vi "DiffIO PWM Disable.vi"(6 "Adapting?":bool, 8 "_SetupElement":T1={"Mode"=enum."Off", "Capture Start [DBTDC]"=0.0, "Capture End [DBTDC]"=0.0, "Polarity"=FALSE, "Frequency [Hz]"=0.0, "Duty Cycle [%]"=0.0, "TDC Offset [CAD]"=0.0, "Window Start [DBTDC]"=0.0, "Window End [DBTDC]"=0.0, "Angles"=[{"Enable"=FALSE, "Location [DBTDC]"=0.0, "Duration [s]"=0.0}, {"Enable"=FALSE, "Location [DBTDC]"=0.0, "Duration [s]"=0.0}, {"Enable"=FALSE, "Location [DBTDC]"=0.0, "Duration [s]"=0.0}, {"Enable"=FALSE, "Location [DBTDC]"=0.0, "Duration [s]"=0.0}], "Skip Fire"=FALSE, "Skip Fire Index"=0} caption="Command Setup" {"Skip Fire Index" max=7; "Angles"."Duration [s]" format="%#_3p"; "Frequency [Hz]" format="%#_3p"}, 11 "Cluster in":refnum<vi>) -> ()   [LabVIEW 2016]
uses:
  Shared/Typedefs/DiffIO-PWM-Settings.ctl
  <vilib>/Powertrain Controls/Device Drivers/DCM/Diff IO/RT/Setup.ctl
  <vilib>/Powertrain Controls/Device Drivers/DCM/Diff IO/FPGA/Mode.ctl
  <vilib>/Powertrain Controls/Device Drivers/DCM/Diff IO/RT/Angle Control.ctl
  <vilib>/Powertrain Controls/Device Drivers/DCM/Diff IO/FPGA/DCM - FPGA - Diff IO.lvlib
  Shared/DSI-Shared.lvlib
  <vilib>/Powertrain Controls/Device Drivers/DCM/Diff IO/RT/DCM - RT - Diff IO.lvlib
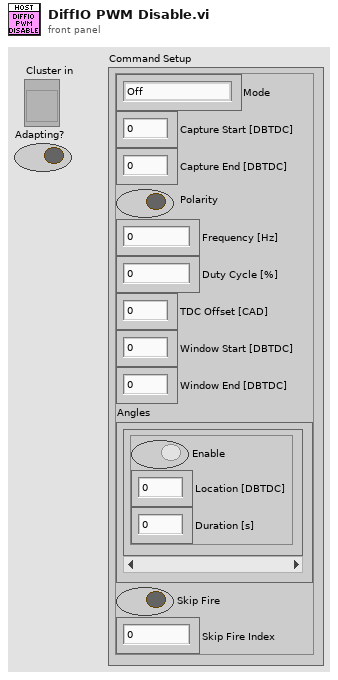
[diagram p1: front panel]
types:
  T1 = typedef "DCM - RT - Diff IO.lvlib/Setup.ctl" = cluster{"Mode":T2, "Capture Start [DBTDC]":sgl, "Capture End [DBTDC]":sgl, "Polarity":bool, "Frequency [Hz]":sgl, "Duty Cycle [%]":sgl, "TDC Offset [CAD]":sgl, "Window Start [DBTDC]":sgl, "Window End [DBTDC]":sgl, "Angles":T3[], "Skip Fire":bool, "Skip Fire Index":u8}
  T2 = typedef "DCM - FPGA - Diff IO.lvlib/Mode.ctl" = enum8{"Off", "Input", "Pulse Width Modulation", "Engine Position Tracking", "Serial Out 1", "Serial Out 2"}
  T3 = typedef "DCM - RT - Diff IO.lvlib/Angle Control.ctl" = cluster{"Enable":bool, "Location [DBTDC]":sgl, "Duration [s]":sgl}
  T4 = enum8{"Enabled", "Disabled", "Disabled and Grayed Out"}
  T5 = typedef "PWM Settings Element.ctl" = cluster{"PWM-TimingMode":enum32{"Frequency", "Period"}, "PWM-Frequency":sgl, "PWM-Period":sgl, "PWM-ControlMode":enum32{"Duty Cycle", "Pulsewidth"}, "PWM-DutyCycle":sgl, "PWM-PulseWidth":sgl}
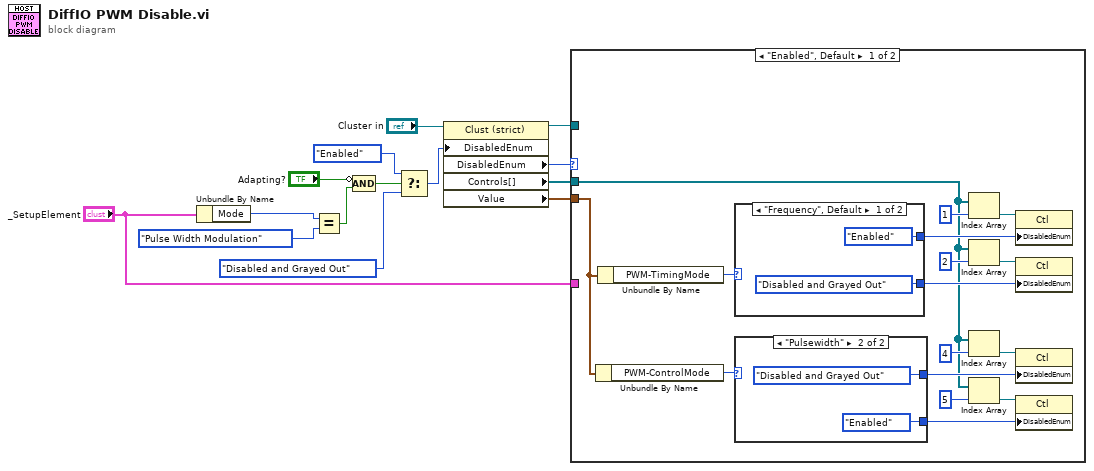
[diagram p0: block diagram]
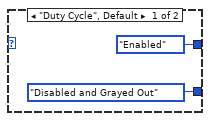
[diagram p2: hidden frame]
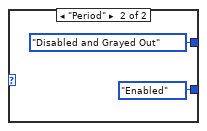
[diagram p3: hidden frame]
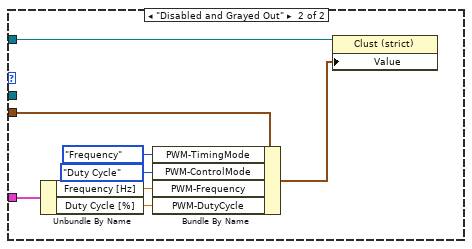
[diagram p4: hidden frame]
diagram:
  n1 = Unbundle By Name("_SetupElement") -> ("Mode"=w2:T2)
  n2 = Equal?(x=w2, y=Mode."Pulse Width Modulation" ("Mode")) -> (x = y?=w5:bool)
  n3 = Compound Arithmetic op=AND(invert "Adapting?", w5) -> (w6:bool)
  n4 = Select(t=T4."Enabled" ("Disabled"), s=w6, f=T4."Disabled and Grayed Out" ("Disabled")) -> (s? t:f=w7:T4)
  n5 = property on="Property Node" class="Clust (strict)"(reference="Cluster in", "DisabledEnum"=w7) -> (reference out=w3:refnum<vi>, "DisabledEnum"=w10:T4, "Controls[]"=w14:refnum<vi>[], "Value"=w13:T5)  [unwired: 1 in, 1 out]
  n6 = case shown="\"Enabled\", Default" w10 {
    tunnel: w13 -> [w24 w45]
    tunnel: w14 -> [w17 _]
    tunnel: w3 -> [_ w46]
    tunnel: "_SetupElement" -> [_ w41]
    frame "Enabled", Default {
      n7 = Unbundle By Name(w24) -> ("PWM-ControlMode"=w25:enum32{"Duty Cycle", "Pulsewidth"})
      n8 = Unbundle By Name(w24) -> ("PWM-TimingMode"=w30:enum32{"Frequency", "Period"})
      n9 = case shown="\"Frequency\", Default" w30 {
        tunnel: [T4."Enabled" ("Disabled") T4."Disabled and Grayed Out" ("Disabled")] -> w29
        tunnel: [T4."Disabled and Grayed Out" ("Disabled") T4."Enabled" ("Disabled")] -> w28
        frame "Frequency", Default {
        }
        frame "Period" {
        }
      }
      n10 = case shown="\"Pulsewidth\"" w25 {
        tunnel: [T4."Enabled" ("Disabled") T4."Disabled and Grayed Out" ("Disabled")] -> w26
        tunnel: [T4."Disabled and Grayed Out" ("Disabled") T4."Enabled" ("Disabled")] -> w27
        frame "Duty Cycle", Default {
        }
        frame "Pulsewidth" {
        }
      }
      n11 = Index Array(array=w17, index=1) -> (element=w21:refnum<vi>)
      n12 = Index Array(array=w17, index=2) -> (element=w20:refnum<vi>)
      n13 = Index Array(array=w17, index=4) -> (element=w16:refnum<vi>)
      n14 = Index Array(array=w17, index=5) -> (element=w15:refnum<vi>)
      n15 = property class="Ctl"(reference=w21, "DisabledEnum"=w29) -> ()  [unwired: 1 in, 2 out]
      n16 = property class="Ctl"(reference=w20, "DisabledEnum"=w28) -> ()  [unwired: 1 in, 2 out]
      n17 = property class="Ctl"(reference=w16, "DisabledEnum"=w26) -> ()  [unwired: 1 in, 2 out]
      n18 = property class="Ctl"(reference=w15, "DisabledEnum"=w27) -> ()  [unwired: 1 in, 2 out]
    }
    frame "Disabled and Grayed Out" {
      n19 = Unbundle By Name(w41) -> ("Frequency [Hz]"=w40:sgl, "Duty Cycle [%]"=w39:sgl)
      n20 = Bundle By Name(cluster=w45, "PWM-TimingMode"=enum32{"Frequency", "Period"}."Frequency", "PWM-ControlMode"=enum32{"Duty Cycle", "Pulsewidth"}."Duty Cycle", "PWM-Frequency"=w40, "PWM-DutyCycle"=w39) -> (w44:T5)
      n21 = property on="Property Node" class="Clust (strict)"(reference=w46, "Value"=w44) -> ()  [unwired: 1 in, 2 out]
    }
  }
